vi "List And Filter Controls From UI.vi"(8 "Error In":errorcluster, 11 "Appearance Actor In":refnum<class "Appearance Actor.lvclass">) -> (0 "Error Out":errorcluster, 3 "Appearance Actor Out":refnum<class "Appearance Actor.lvclass">)   [LabVIEW 2021, in "Appearance Actor.lvlib" / "Appearance Actor.lvclass"]
uses:
  Appearance Actor.lvclass
  Appearance Actor.lvclass/Appearance Actor.ctl
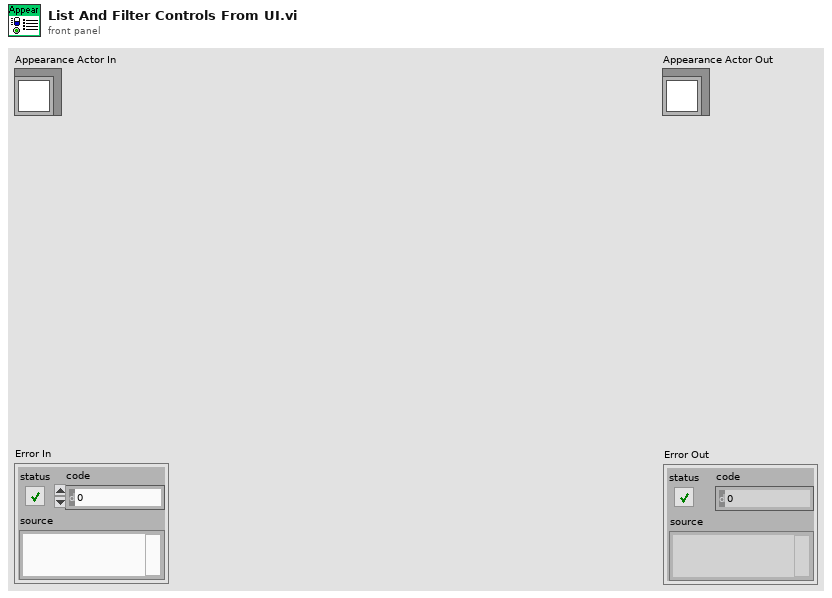
[diagram p1: front panel]
types:
  T1 = typedef "Appearance Actor.lvlib/Appearance Actor.lvclass/UI Controls--map.ctl" = map{string, T2}
  T2 = typedef "Appearance Actor.lvlib/Appearance Actor.lvclass/Element Controls--map.ctl" = map{string, T3}
  T3 = typedef "Appearance Actor.lvlib/Appearance Actor.lvclass/Controls--map.ctl" = map{string, refnum<vi>}
  T4 = typedef "Appearance Actor.lvlib/Appearance Actor.lvclass/UI Panes--map.ctl" = map{string, T5}
  T5 = typedef "Appearance Actor.lvlib/Appearance Actor.lvclass/Element Panes--map.ctl" = map{string, T6}
  T6 = typedef "Appearance Actor.lvlib/Appearance Actor.lvclass/Panes--map.ctl" = map{string, refnum<vi>}
  T7 = typedef "Appearance Actor.lvlib/Appearance Actor.lvclass/UI Splitters--map.ctl" = map{string, T8}
  T8 = typedef "Appearance Actor.lvlib/Appearance Actor.lvclass/Element Splitters--map.ctl" = map{string, T9}
  T9 = typedef "Appearance Actor.lvlib/Appearance Actor.lvclass/Splitters--map.ctl" = map{string, refnum<vi>}
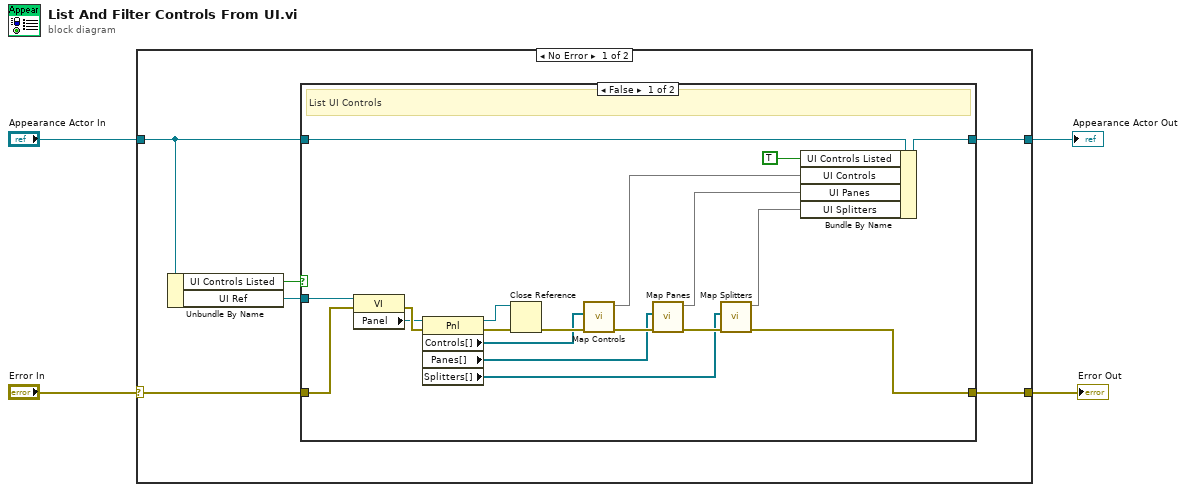
[diagram p0: block diagram]
diagram:
  n1 = case shown="No Error" "Error In" {
    selector: "Error In" -> [w10 w33]
    tunnel: [w8 w33] -> w3
    tunnel: "Appearance Actor In" -> [w7 w32]
    tunnel: [w9 w32] -> w1
    frame No Error {
      n2 = Unbundle By Name(w7) -> ("UI Controls Listed"=w6:bool, "UI Ref"=w5:refnum<vi>)
      n3 = case shown="False" w6 {
        tunnel: w5 -> [w29 _]
        tunnel: w10 -> [w27 w30]
        tunnel: w7 -> [w23 w31]
        tunnel: [w22 w31] -> w9
        tunnel: [w11 w30] -> w8
        frame False {
          # "List UI Controls"
          n4 = property class="VI"(reference=w29, error in=w27) -> (error out=w26:errorcluster, "Panel"=w25:refnum<vi>)  [unwired: 1 out]
          n5 = property class="Pnl"(reference=w25, error in=w26) -> (reference out=w28:refnum<vi>, error out=w24:errorcluster, "Controls[]"=w17:refnum<vi>[], "Panes[]"=w16:refnum<vi>[], "Splitters[]"=w15:refnum<vi>[])
          n6 = Close Reference(reference=w28, error in (no error)=w24) -> (error out=w20:errorcluster)
          n7 = call "Map Controls.vi"("Error In"=w20, "Control Refs"=w17) -> ("Error Out"=w19:errorcluster, "UI Controls Out"=w14:T1)  [unwired: 8 in]
          n8 = call "Map Panes.vi"("Error In"=w19, "Control Refs"=w16) -> ("Error Out"=w18:errorcluster, "UI Panes Out"=w13:T4)  [unwired: 8 in]
          n9 = call "Map Splitters.vi"("Error In"=w18, "Control Refs"=w15) -> ("Error Out"=w11:errorcluster, "UI Splitters Out"=w12:T7)  [unwired: 8 in]
          n10 = Bundle By Name(cluster=w23, "UI Controls Listed"=TRUE ("UI Controls Registered"), "UI Controls"=w14, "UI Panes"=w13, "UI Splitters"=w12) -> (w22:refnum<class "Appearance Actor.lvclass">)
        }
        frame True {
          # "UI Controls Already Listed, Do Nothing"
        }
      }
    }
    frame Error {
    }
  }
  "Error Out" <- w3
  "Appearance Actor Out" <- w1
